vi "act-19- gestion de stock.vi"() -> ()   [LabVIEW 2010]
uses:
  act/lv_07/lv_07.lvlib
panel:
  out "Qe":dbl
  in  "Pu":dbl
  in  "Qa":dbl
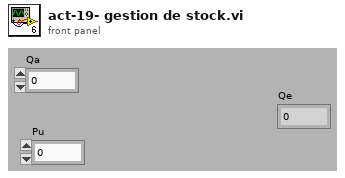
[diagram p1: front panel]
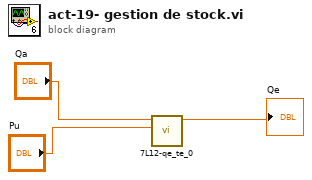
[diagram p0: block diagram]
diagram:
  n1 = call "7L12-qe_te_0.vi"("Pu"="Pu", "Qa"="Qa") -> ("Qe"=→"Qe":dbl)  [unwired: 7 in, 2 out]
